vi "Write Module.vi"(5 "Channel Type":T5, 7 "R/W Case":T4, 8 "error in (no error)":errorcluster, 9 "Input FIFO buffer in":dbl[](array[numeric]), 10 "Input Data in":T1 {"BD Refs"."Data Reference" format="%.0x"}, 11 "IOV ref in":T6) -> (0 "error out":errorcluster, 1 "Input FIFO buffer out":dbl[](array[numeric]), 2 "Input Data out":T1 {"BD Refs"."Data Reference" format="%.0x"}, 3 "IOV ref out":T6)   [LabVIEW 2020, in "SEECD Engine.lvlib"]
uses:
  SEECD Engine.lvlib
  <vilib>/NI VeriStand/Custom Device API/Custom Device API.lvlib
  <vilib>/NI VeriStand/Custom Device API/Data Reference.ctl
  <vilib>/NI VeriStand/Custom Device API/Block Data Reference.ctl
  Includes/Modules.lvlibp/RSI Module/Channel Type.ctl
  Type Defs/RW Case.ctl
  Type Defs/Input Data.ctl
  Type Defs/Open Module IOVs.ctl
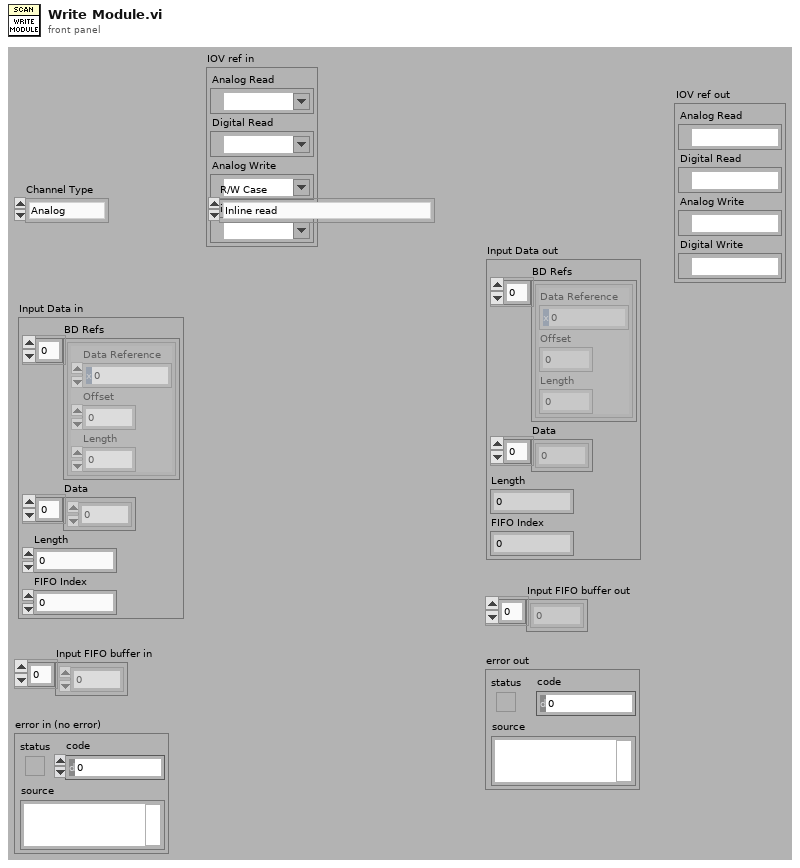
[diagram p1: front panel]
types:
  T1 = typedef "SEECD Engine.lvlib/Input Data.ctl" = cluster{"BD Refs":T2[], "Data":dbl[], "Length":i32, "FIFO Index":i32}
  T2 = typedef "Custom Device API.lvlib/Block Data Reference.ctl" = cluster{"Data Reference":T3, "Offset":u64, "Length":u64}
  T3 = typedef "Custom Device API.lvlib/Data Reference.ctl" = i32
  T4 = typedef "SEECD Engine.lvlib/RW Case.ctl" = enum16{"Inline read", "Inline write", "Async - Inline loop read", "Async - Inline loop write", "Async loop (read/write)"}
  T5 = typedef "Modules.lvlibp/RSI Module.lvclass/Channel Type.ctl" = enum16{"Analog", "Digital"}
  T6 = typedef "SEECD Engine.lvlib/Open Module IOVs.ctl" = cluster{"Analog Read":refnum<k21>, "Digital Read":refnum<k21>, "Analog Write":refnum<k21>, "Digital Write":refnum<k21>}
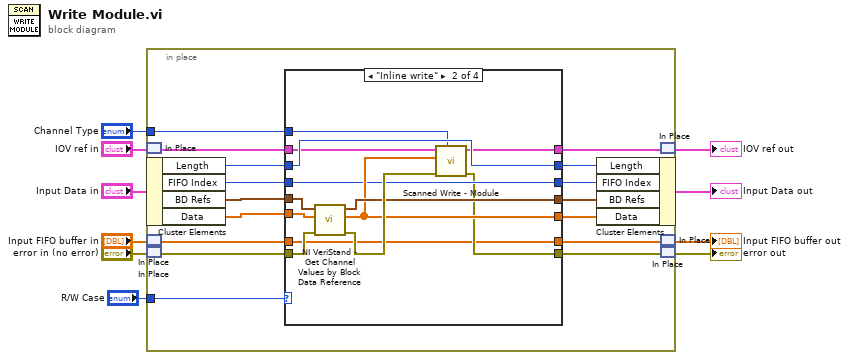
[diagram p0: block diagram]
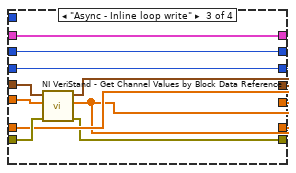
[diagram p3: hidden frame]
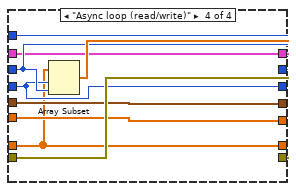
[diagram p4: hidden frame]
diagram:
  n1 = in-place {
    in-place-border: "R/W Case" -> [w26]
    in-place-border: "Channel Type" -> [w25]
    n2 = in-place-match #1("IOV ref in") -> (w16:T6)
    n3 = in-place-cluster #2("Input Data in") -> ("Length"=w19:i32, "FIFO Index"=w22:i32, "BD Refs"=w11:T2[], "Data"=w12:dbl[])
    n4 = in-place-match #3("Input FIFO buffer in") -> (w18:dbl[])
    n5 = in-place-match #4("error in (no error)") -> (w14:errorcluster)
    n6 = case shown="\"Inline write\"" w26 {
      tunnel: w14 -> [w27 w46 w57 w68]
      tunnel: w18 -> [w28 w36 w54 w58]
      tunnel: w19 -> [w31 w42 w51 w64]
      tunnel: w22 -> [w32 w41 w50 w63]
      tunnel: w11 -> [w30 w34 w56 w66]
      tunnel: w12 -> [w29 w35 w55 w67]
      tunnel: [w29 w43 w52 w67] -> w23
      tunnel: [w30 w44 w53 w66] -> w24
      tunnel: [w31 w42 w51 w64] -> w20
      tunnel: [w32 w41 w50 w63] -> w21
      tunnel: [w33 w40 w49 w62] -> w15
      tunnel: w16 -> [w33 w39 w49 w61]
      tunnel: w25 -> [_ w38 _ w60]
      tunnel: [w27 w37 w48 w59] -> w13
      tunnel: [w28 w36 w47 w58] -> w17
      frame Default {
      }
      frame "Inline write" {
        n7 = call <vilib>:"NI VeriStand - Get Channel Values by Block Data Reference.vi"("error in (no error)"=w46, "Values Array in"=w35, "Block Data Ref"=w34) -> ("error out"=w45:errorcluster, "Values Array out"=w43:dbl[], "Block Data Ref dup"=w44:T2[])  [unwired: 6 in]
        n8 = call "Scanned Write - Module.vi"("Channel Type"=w38, "error in (no error)"=w45, "data in"=w43, "IOV ref in"=w39) -> ("error out"=w37:errorcluster, "IOV ref out"=w40:T6)  [unwired: 5 in]
      }
      frame "Async - Inline loop write" {
        n9 = call <vilib>:"NI VeriStand - Get Channel Values by Block Data Reference.vi"("error in (no error)"=w57, "Values Array in"=w55, "Block Data Ref"=w56) -> ("error out"=w48:errorcluster, "Values Array out"=w52:dbl[], "Block Data Ref dup"=w53:T2[])  [unwired: 6 in]
        n10 = Replace Array Subset(array=w54, new element=w52, index=w50) -> (w47:dbl[])
      }
      frame "Async loop (read/write)" {
        n11 = Array Subset(array=w58, index=w63, length=w64) -> (w65:dbl[])
        n12 = call "Scanned Write - Module.vi"("Channel Type"=w60, "error in (no error)"=w68, "data in"=w65, "IOV ref in"=w61) -> ("error out"=w59:errorcluster, "IOV ref out"=w62:T6)  [unwired: 5 in]
      }
    }
    n13 = in-place-cluster #2("Length"=w20, "FIFO Index"=w21, "BD Refs"=w24, "Data"=w23) -> (→"Input Data out":T1)
    n14 = in-place-match #1(w15) -> (→"IOV ref out":T6)
    n15 = in-place-match #3(w17) -> (→"Input FIFO buffer out":dbl[])
    n16 = in-place-match #4(w13) -> (→"error out":errorcluster)
  }
